vi "M9290A Init.vi"(8 "error in":errorcluster, 11 "SpecAn Ref In":refnum<visa-resource-name>) -> (0 "error out":errorcluster, 3 "SpecAn Ref Out":refnum<visa-resource-name>)   [LabVIEW 2015]
uses:
  <instrlib>/Agilent MXA Series/Public/Configure/Trigger/Configure Trigger (Normal).vi
  <instrlib>/Agilent MXA Series/Agilent MXA Series.lvlib
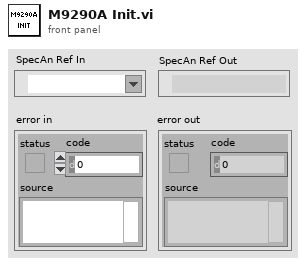
[diagram p1: front panel]
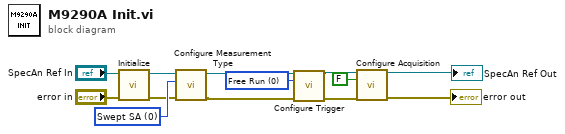
[diagram p0: block diagram]
diagram:
  w6 = 0 items=["Free Run", "Video", "Line", "External1", "External2", "RF Burst"] ("Trigger Source (0: Free Run)")
  w11 = 0 items=["Swept SA", "Channel Power", "Occupied Bandwidth", "Power Stat CCDF", "Adjacent Channel Power", "Burst Power", "Spurious Emissions", "Spectrum Emission Mask", "List Sweep", "TOI", "Harmonic"] ("Measurement Type (0: Swept SA)")
  n1 = call <instrlib>:"Initialize.vi"("error in (no error)"="error in", "VISA resource name"="SpecAn Ref In") -> ("error out"=w9:errorcluster, "VISA resource name out"=w10:refnum<visa-resource-name>)  [unwired: 8 in]
  n2 = call <instrlib>:"Configure Measurement Type.vi"("error in (no error)"=w9, "Measurement Type (0: Swept SA)"=w11, "VISA resource name"=w10) -> ("error out"=w2:errorcluster, "VISA resource name out"=w1:refnum<visa-resource-name>)  [unwired: 7 in]
  n3 = call-poly <instrlib>:"Configure Trigger.vi"("VISA resource name"=w1, "Trigger Source (0: Free Run)"=w6, "error in (no error)"=w2) -> ("VISA resource name out"=w8:refnum<visa-resource-name>, "error out"=w7:errorcluster)  [unwired: 11 in]
  n4 = call <instrlib>:"Configure Acquisition.vi"("VISA resource name"=w8, "Enable Continuous Sweep (T: Enable)"=FALSE, "error in (no error)"=w7) -> ("VISA resource name out"=→"SpecAn Ref Out":refnum<visa-resource-name>, "error out"=→"error out":errorcluster)  [unwired: 11 in]
